vi "Get Alias.vi"(8 "error in (no error)":errorcluster, 10 "Alias":string, 11 "Aliases Ref in":T1 format="%.0x") -> (0 "error out":errorcluster, 1 "Alias found":bool, 2 "Pin":string, 3 "Aliases Ref out":T1 format="%.0x")   [LabVIEW 2017, in "Switch Scripting.lvlib"]
uses:
  Switch Scripting.lvlib
  <vilib>/NI Veristand/Custom Device API/Custom Device Item Ref.ctl
  <vilib>/NI Veristand/Custom Device API/Get Item Property (String).vi
  <vilib>/NI VeriStand/Custom Device API/Custom Device API.lvlib
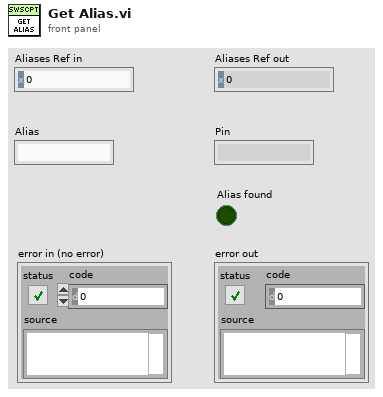
[diagram p1: front panel]
types:
  T1 = typedef "Custom Device API.lvlib/Custom Device Item Ref.ctl" = u64
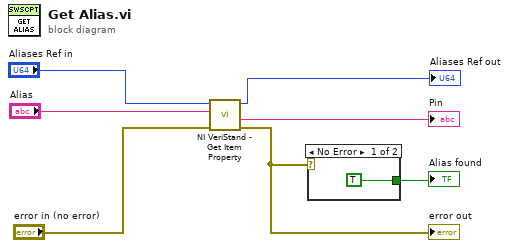
[diagram p0: block diagram]
diagram:
  n1 = call-poly <vilib>:"NI VeriStand - Get Item Property.vi"("error in (no error)"="error in (no error)", "Property Name"="Alias", "Item Ref in"="Aliases Ref in") -> ("error out"=w1:errorcluster, "Value"=→"Pin":string, "Item Ref out"=→"Aliases Ref out":T1)  [unwired: 5 in, 1 out]
  "error out" <- w1
  n2 = case shown="No Error" w1 {
    tunnel: [TRUE ("Alias found") _] -> w3
    frame No Error {
    }
    frame Error {
    }
  }
  "Alias found" <- w3
